vi "read vectornav.vi"() -> ()   [LabVIEW 2009]
uses:
  <vilib>/Instr/_visa.llb/VISA Configure Serial Port (Instr).vi
  Athena Localization Data.vi
  vectornav data.vi
  UDP3-GPS, INS/UDP3rtglob.vi
panel:
  out "x*y":dbl
  in  "VISA resource name":refnum<visa-resource-name>="ASRL1::INSTR"
  out "z-magnetic":dbl
  out "y-magnetic":dbl
  out "x-magnetic":dbl
  out "y-acceleration 2":dbl
  out "y-acceleration":dbl
  out "x-acceleration":dbl
  out "q[3]":dbl
  out "q[2]":dbl
  out "q[1]":dbl
  out "q[0]":dbl
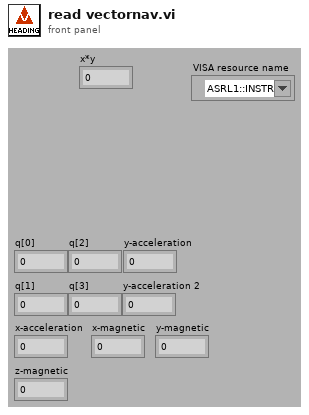
[diagram p1: front panel]
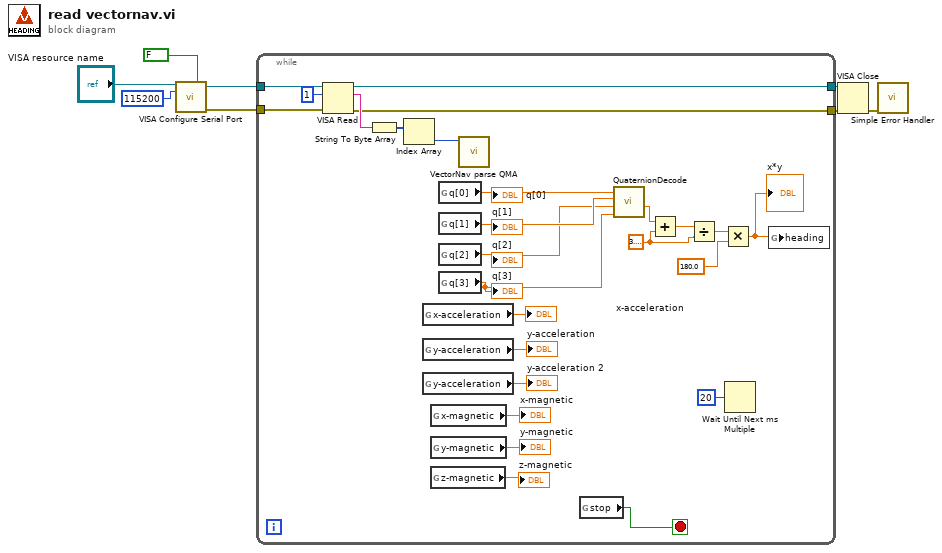
[diagram p0: block diagram]
diagram:
  n1 = call-poly "VISA Configure Serial Port"("VISA resource name"="VISA resource name", "Enable Termination\nChar (T)"=FALSE ("Enable Termination\nChar (T)"), "baud rate (9600)"=u32 115200) -> ("VISA resource name out"=w4:refnum<visa-resource-name>, "error out"=w5:errorcluster)  [unwired: 11 in]
  n2 = while {
    tunnel: w5 -> [w25]
    tunnel: w4 -> [w24]
    tunnel: [w22] -> w3
    tunnel: [w21] -> w2
    stop <- w9 stop-if-true
    w14 = 3.141592653589793
    n3 = VISA Read(VISA resource name=w24, byte count=u32 1, error in (no error)=w25) -> (VISA resource name out=w22:refnum<visa-resource-name>, read buffer=w28:string, error out=w21:errorcluster)  [unwired: 1 out]
    n4 = String To Byte Array(string=w28) -> (unsigned byte array=w27:u8[])
    n5 = Index Array(array=w27) -> (element=w26:u8)  [unwired: 1 in]
    n6 = global read "vectornav data.vi" "x-acceleration"() -> (→"x-acceleration":dbl)
    n7 = global read "vectornav data.vi" "y-acceleration"() -> (→"y-acceleration":dbl)
    n8 = global read "vectornav data.vi" "y-acceleration"() -> (→"y-acceleration 2":dbl)
    n9 = global read "vectornav data.vi" "x-magnetic"() -> (→"x-magnetic":dbl)
    n10 = global read "vectornav data.vi" "y-magnetic"() -> (→"y-magnetic":dbl)
    n11 = global read "vectornav data.vi" "z-magnetic"() -> (→"z-magnetic":dbl)
    n12 = global read "vectornav data.vi" "q[0]"() -> (w20:dbl)
    "q[0]" <- w20
    n13 = global read "vectornav data.vi" "q[1]"() -> (w19:dbl)
    "q[1]" <- w19
    n14 = global read "vectornav data.vi" "q[2]"() -> (w18:dbl)
    "q[2]" <- w18
    n15 = global read "vectornav data.vi" "q[3]"() -> (w17:dbl)
    "q[3]" <- w17
    n16 = call "VectorNav parse QMA.vi"("input data"=w26) -> ()  [unwired: 11 in]
    n17 = global read "UDP3rtglob.vi" "stop"() -> (w9:bool)
    n18 = call "QuaternionDecode.vi"("qw"=w17, "qz"=w18, "qy"=w19, "qx"=w20) -> ("heading"=w16:dbl)  [unwired: 7 in]
    n19 = Add(x=w16, y=w14) -> (x+y=w15:dbl)
    n20 = Divide(x=w15, y=w14) -> (x/y=w13:dbl)
    n21 = Multiply(x=w13, y=180.0) -> (x*y=w11:dbl)
    "x*y" <- w11
    n22 = Wait Until Next ms Multiple(millisecond multiple=u32 20) -> ()  [unwired: 1 out]
    n23 = global write "Athena Localization Data.vi" "heading"(w11) -> ()
  }
  n24 = VISA Close(VISA resource name=w3, error in (no error)=w2) -> (error out=w1:errorcluster)
  n25 = call <vilib>:"Simple Error Handler.vi"("error in (no error)"=w1) -> ()  [unwired: 4 in, 5 out]
